vi "Write Exception Status.vi"(8 "error in (no error)":errorcluster, 10 "exception status":u8 format="%02x", 11 "device data model in":refnum<class "WebSocket Data Model.lvclass">) -> (0 "error out":errorcluster, 3 "device data model out":refnum<class "WebSocket Data Model.lvclass">)   [LabVIEW 2021, in "WebSockets.lvlib" / "WebSocket Data Model.lvclass"]
doc: "Sets the exception status in the device data model."
uses:
  WebSocket Data Model.lvclass
  WebSocket Data Model.lvclass/WebSocket Data Model.ctl
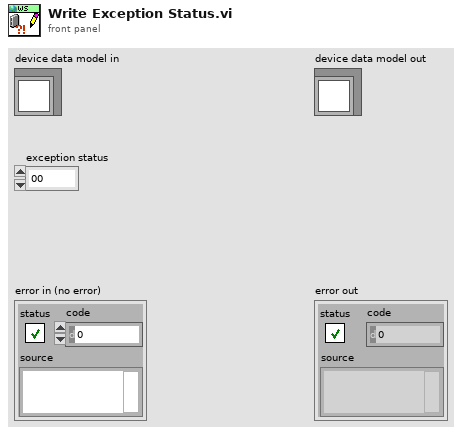
[diagram p1: front panel]
types:
  T1 = typedef "WebSockets.lvlib/WebSocket Data Model.lvclass/Data Model.ctl" = cluster{"UTC":u64, "Receive Binary Data":u8[], "Receive Text Data":string, "Send Binary Data":u8[], "Send Text Data":string, "ES":u8}
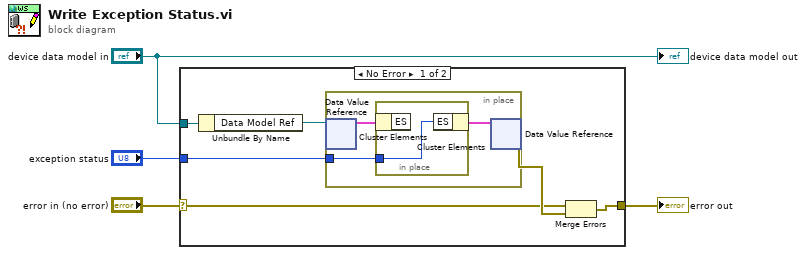
[diagram p0: block diagram]
diagram:
  n1 = case shown="No Error" "error in (no error)" {
    selector: "error in (no error)" -> [w5 w15]
    tunnel: [w10 w15] -> w4
    tunnel: "device data model in" -> [w9 _]
    tunnel: "exception status" -> [w8 _]
    frame No Error {
      n2 = Unbundle By Name(w9) -> ("Data Model Ref"=w7:refnum<data-value>)
      n3 = in-place {
        in-place-border: w8 -> [w12]
        n4 = in-place-dvr #1(w7) -> (w13:T1)  [unwired: 1 out]
        n5 = in-place {
          in-place-border: w12 -> [w14]
          n6 = in-place-cluster #2(w13) -> ()  [unwired: 1 out]
          n7 = in-place-cluster #2("ES"=w14) -> (w11:T1)
        }
        n8 = in-place-dvr #1(w11) -> (w6:errorcluster)  [unwired: 1 out]
      }
      n9 = Merge Errors(w5, w6) -> (w10:errorcluster)
    }
    frame Error {
    }
  }
  "error out" <- w4
  "device data model out" <- "device data model in"
